vi "ge_CheckQsClosed.vi"(8 "error in":errorcluster, 9 "Timeout(ms)":u32=1000, 11 "All DAQ Processes":T1[](array[typedef])) -> (0 "error out":errorcluster)   [LabVIEW 2012]
uses:
  SubVIs DAQ/Custom Ctrls/ge_QName and Ref.ctl
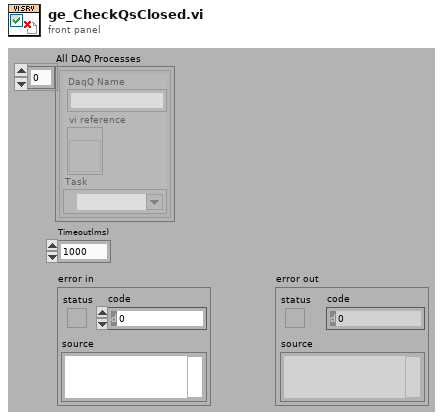
[diagram p1: front panel]
types:
  T1 = typedef "ge_QName and Ref.ctl" = cluster{"DaqQ Name":string, "vi reference":refnum<vi>, "Task":refnum<k21>}
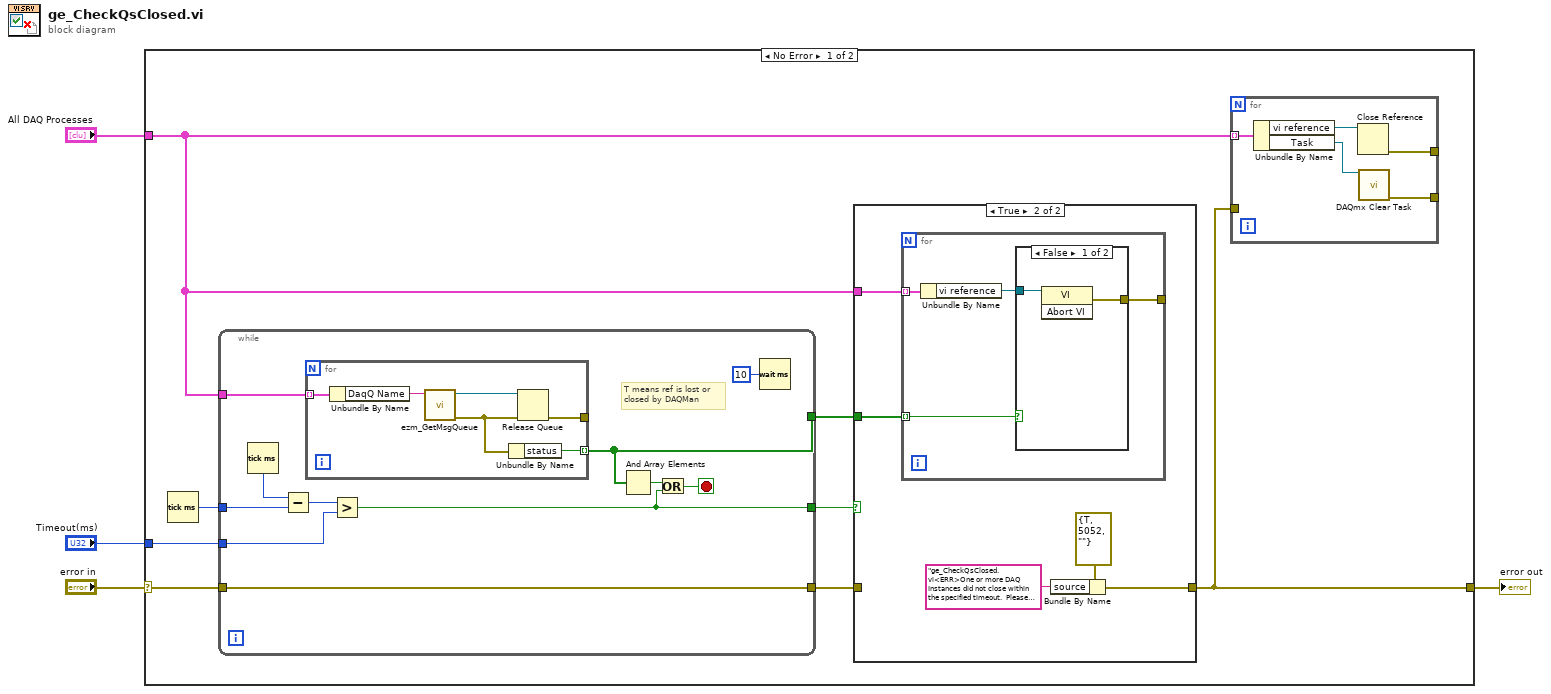
[diagram p0: block diagram]
diagram:
  n1 = case shown="No Error" "error in" {
    selector: "error in" -> [w10 w48]
    tunnel: "Timeout(ms)" -> [w12 _]
    tunnel: [w5 w48] -> w2
    tunnel: "All DAQ Processes" -> [w6 _]
    frame No Error {
      n2 = Tick Count (ms)() -> (millisecond timer value=w11:u32)
      n3 = while {
        tunnel: w12 -> [w38]
        tunnel: w10 -> [w36]
        tunnel: [w36] -> w7
        tunnel: [w35] -> w8
        tunnel: w11 -> [w40]
        tunnel: [w32] -> w9
        tunnel: w6 -> [w31]
        stop <- w37 stop-if-true
        # "T means ref is lost or\nclosed by DAQMan"
        n4 = Tick Count (ms)() -> (millisecond timer value=w41:u32)
        n5 = Subtract(x=w41, y=w40) -> (x-y=w39:u32)
        n6 = for {
          tunnel: w31 -> [w46] mode=indexing
          tunnel: [w45] -> w32 mode=indexing
          tunnel: [w42] -> _
          n7 = Unbundle By Name(w46) -> ("DaqQ Name"=w47:string)
          n8 = call "ezm_GetMsgQueue.vi"("Queue Name"=w47) -> ("error out"=w43:errorcluster, "queue out"=w44:refnum<queue>)  [unwired: 9 in]
          n9 = Unbundle By Name(w43) -> ("status"=w45:bool)
          n10 = Release Queue(queue=w44, error in (no error)=w43) -> (error out=w42:errorcluster)  [unwired: 1 in, 2 out]
        }
        n11 = Greater?(x=w39, y=w38) -> (0:w35:bool)
        n12 = And Array Elements(Boolean array=w32) -> (logical AND=w33:bool)
        n13 = Or(x=w33, y=w35) -> (x .or. y?=w37:bool)
        n14 = Wait (ms)(milliseconds to wait=u32 10) -> ()  [unwired: 1 out]
      }
      n15 = case shown="True" w8 {
        tunnel: w6 -> [_ w23]
        tunnel: w9 -> [_ w22]
        tunnel: w7 -> [w18 _]
        tunnel: [w18 w19] -> w5
        frame False {
        }
        frame True {
          n16 = for {
            tunnel: w23 -> [w26] mode=indexing
            tunnel: w22 -> [w27] mode=indexing
            tunnel: [w24] -> _
            n17 = Unbundle By Name(w26) -> ("vi reference"=w25:refnum<vi>)
            n18 = case shown="False" w27 {
              tunnel: w25 -> [w29 _]
              tunnel: [w28 errorcluster {"status"=FALSE, "code"=0, "source"=""} ("error out")] -> w24
              frame False {
                n19 = invoke class="VI" method="Abort VI"(reference=w29) -> (error out=w28:errorcluster)  [unwired: 2 in, 2 out]
              }
              frame True {
              }
            }
          }
          n20 = Bundle By Name(cluster=errorcluster {"status"=TRUE, "code"=5052, "source"=""} ("error IO"), "source"="ge_CheckQsClosed.vi<ERR>One or more DAQ Instances did not close within the specified timeout.  Please restart the application. ") -> (w19:errorcluster)
        }
      }
      n21 = for {
        tunnel: w6 -> [w17] mode=indexing
        tunnel: w5 -> [_]
        tunnel: [w14] -> _
        tunnel: [w13] -> _
        n22 = Unbundle By Name(w17) -> ("vi reference"=w16:refnum<vi>, "Task"=w15:refnum<k21>)
        n23 = Close Reference(reference=w16) -> (error out=w14:errorcluster)  [unwired: 1 in]
        n24 = call <vilib>:"DAQmx Clear Task.vi"("task in"=w15) -> ("error out"=w13:errorcluster)  [unwired: 14 in]
      }
    }
    frame Error {
    }
  }
  "error out" <- w2
